vi "vector 2 cluster.vi"(1 "coordinates":dbl[][](array[numeric]) format="%.2f") -> (0 "?":cluster{"x":dbl[], "y":dbl[]} {"y" format="%.2f"; "x" format="%.2f"})   [LabVIEW 2019]
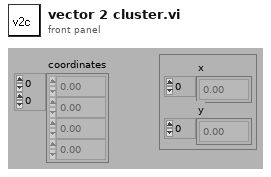
[diagram p1: front panel]
types:
  T1 = cluster{"coordinates":dbl[], "coordinates":dbl[]}
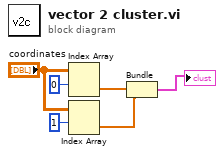
[diagram p0: block diagram]
diagram:
  n1 = Index Array(array="coordinates", index (row)=0) -> (element=w4:dbl[])  [unwired: 1 in]
  n2 = Index Array(array="coordinates", index (row)=1) -> (element=w5:dbl[])  [unwired: 1 in]
  n3 = Bundle("coordinates"=w4, "coordinates"=w5) -> (→"?":T1)  [unwired: 1 out]
